vi "Logging Loop.vi"(5 "Acquisition and Logging":refnum<queue>, 7 "Message Handler":refnum<queue>, 8 "FIFO Cluster":T1, 9 "Name Cluster":T2, 10 "Ready to log":refnum<vi>, 11 "Logging Cluster":refnum<vi>) -> ()   [LabVIEW 2017]
uses:
  Controls/Logging names.ctl
  Message Queue/Message Cluster.ctl
  Message Queue/Message Queue.lvlib
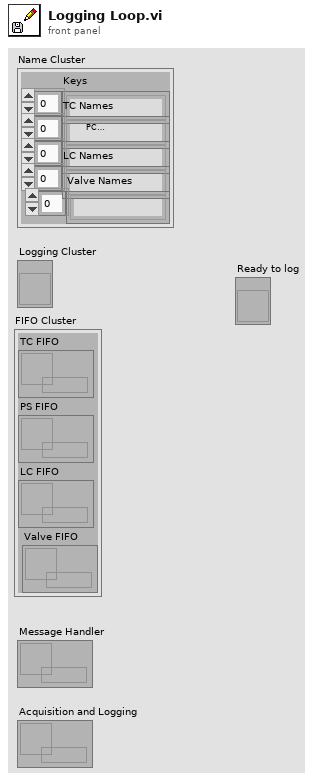
[diagram p1: front panel]
types:
  T1 = cluster{"TC FIFO":refnum<k33>, "PS FIFO":refnum<k33>, "LC FIFO":refnum<k33>, "Valve FIFO":refnum<k33>}
  T2 = typedef "Logging names.ctl" = cluster{"Keys":string[], "TC Names":string[], "PC Names":string[], "LC Names":string[], "Valve Names":string[]}
  T3 = cluster{"TC Logging":cluster{"TC 1":bool, "TC 2":bool, "TC 3":bool, "TC 4":bool, "TC 5":bool, "TC 6":bool, "TC 7":bool, "TC 8":bool, "TC 9":bool, "TC 10":bool, "TC 11":bool, "TC 12":bool, "TC 13":bool, "TC 14":bool, "TC 15":bool, "TC 16":bool}, "PS Logging":cluster{"PS 1":bool, "PS 2":bool, "PS 3":bool, "PS 4":bool, "PS 5":bool, "PS 6":bool, "PS 7":bool, "PS 8":bool}, "LC Logging":cluster{"LC 1":bool, "LC 2":bool, "LC 3":bool, "LC 4":bool}}
  T4 = enum16{"open", "open or create", "create or replace", "create", "open (read-only)"}
  T5 = typedef "Logging Settings.ctl" = cluster{"Logging Channels":cluster{"TC Logging":cluster{"TC 1":bool, "TC 2":bool, "TC 3":bool, "TC 4":bool, "TC 5":bool, "TC 6":bool, "TC 7":bool, "TC 8":bool, "TC 9":bool, "TC 10":bool, "TC 11":bool, "TC 12":bool, "TC 13":bool, "TC 14":bool, "TC 15":bool, "TC 16":bool}, "PS Logging":cluster{"PS 1":bool, "PS 2":bool, "PS 3":bool, "PS 4":bool, "PS 5":bool, "PS 6":bool, "PS 7":bool, "PS 8":bool}, "LC Logging":cluster{"LC 1":bool, "LC 2":bool, "LC 3":bool, "LC 4":bool}}, "TC Low Speed Logging":u32, "TC  High Speed Logging":u32, "PS Low Speed Logging":u32, "PS  High Speed Logging":u32, "LC Low Speed Logging":u32, "LC  High Speed Logging":u32, "Valve Names":string[]}
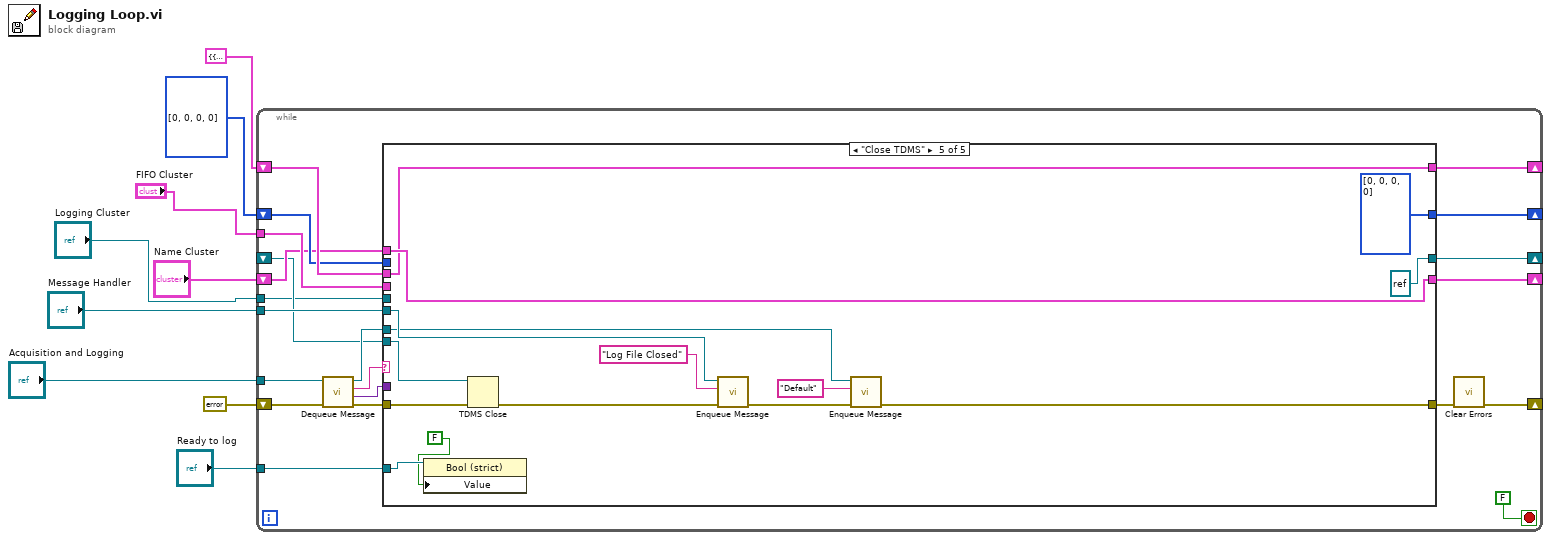
[diagram p0: block diagram]
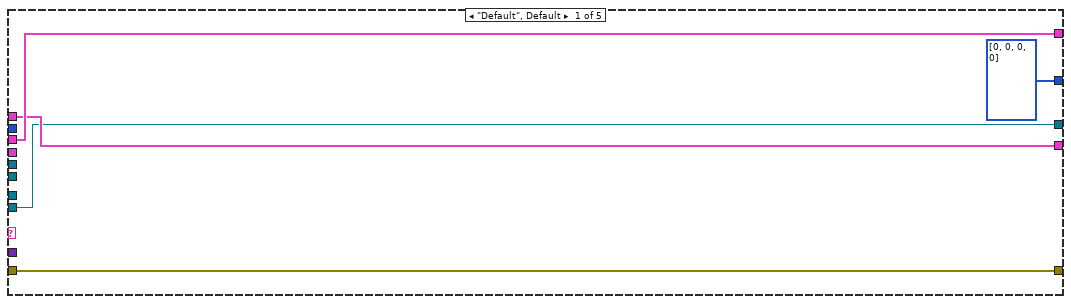
[diagram p2: hidden frame]
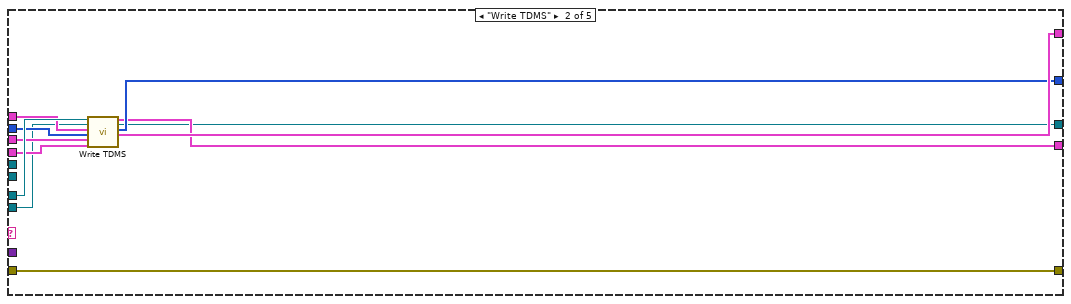
[diagram p3: hidden frame]
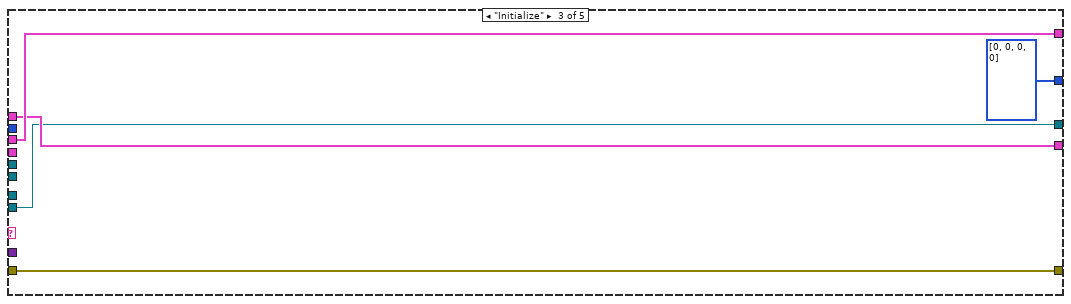
[diagram p4: hidden frame]
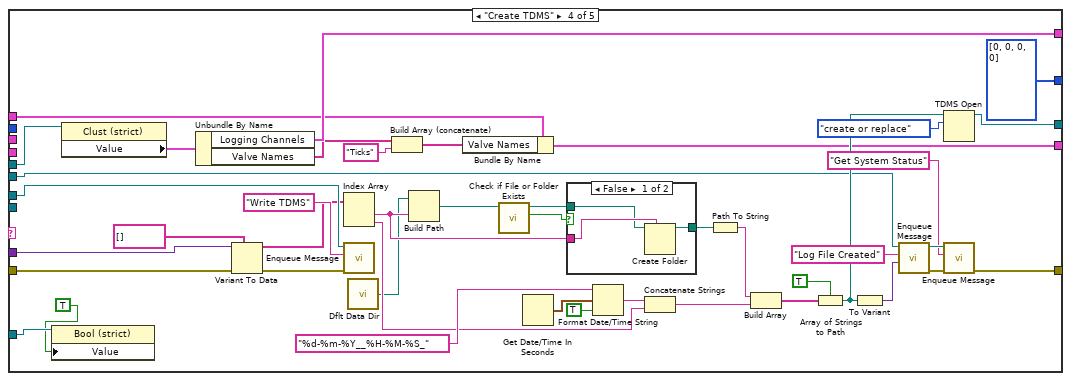
[diagram p5: hidden frame]
diagram:
  n1 = while {
    tunnel: "Acquisition and Logging" -> [w30]
    shift-right: [w18] -> _
    shift-left: errorcluster {"status"=FALSE, "code"=0, "source"=""} ("error out") -> [w24]
    tunnel: "FIFO Cluster" -> [w22]
    tunnel: "Message Handler" -> [w21]
    shift-right: [w20] -> _
    shift-left: T3 {"TC Logging"={"TC 1"=FALSE, "TC 2"=FALSE, "TC 3"=FALSE, "TC 4"=FALSE, "TC 5"=FALSE, "TC 6"=FALSE, "TC 7"=FALSE, "TC 8"=FALSE, "TC 9"=FALSE, "TC 10"=FALSE, "TC 11"=FALSE, "TC 12"=FALSE, "TC 13"=FALSE, "TC 14"=FALSE, "TC 15"=FALSE, "TC 16"=FALSE}, "PS Logging"={"PS 1"=FALSE, "PS 2"=FALSE, "PS 3"=FALSE, "PS 4"=FALSE, "PS 5"=FALSE, "PS 6"=FALSE, "PS 7"=FALSE, "PS 8"=FALSE}, "LC Logging"={"LC 1"=FALSE, "LC 2"=FALSE, "LC 3"=FALSE, "LC 4"=FALSE}} ("Logging Channels") -> [w19]
    shift-right: [w16] -> _
    shift-left: u32[] [0, 0, 0, 0] -> [w17]
    shift-right: [w15] -> _
    shift-left: "Name Cluster" -> [w14]
    shift-right: [w13] -> _
    shift-left: _ -> [w12]
    tunnel: "Logging Cluster" -> [w11]
    tunnel: "Ready to log" -> [w10]
    stop <- FALSE stop-if-true
    n2 = call "Dequeue Message.vi"("error in (no error)"=w24, "Message Queue"=w30) -> ("error out"=w29:errorcluster, "Message Data"=w27:variant, "Message"=w26:string, "dup Message Queue"=w28:refnum<queue>)  [unwired: 6 in]
    n3 = case shown="\"Close TDMS\"" w26 {
      tunnel: w29 -> [w35 w46 w48 w81 w113]
      tunnel: w28 -> [_ w45 _ w89 w104]
      tunnel: w27 -> [_ _ _ w82 _]
      tunnel: [w35 w46 w48 w66 w105] -> w23
      tunnel: w22 -> [_ w43 _ _ _]
      tunnel: w14 -> [w32 w44 w49 w76 w112]
      tunnel: w21 -> [_ _ _ w69 w109]
      tunnel: [w34 w40 w51 w84 w111] -> w20
      tunnel: w19 -> [w34 w42 w51 _ w111]
      tunnel: w17 -> [_ w41 _ _ _]
      tunnel: [u32[] [0, 0, 0, 0] w39 u32[] [0, 0, 0, 0] u32[] [0, 0, 0, 0] u32[] [0, 0, 0, 0]] -> w16
      tunnel: [w32 w38 w49 w73 w112] -> w15
      tunnel: [w31 w37 w47 w65 refnum<k34> refnum ("tdms file out")] -> w13
      tunnel: w12 -> [w31 w36 w47 _ w101]
      tunnel: w11 -> [_ _ _ w64 _]
      tunnel: w10 -> [_ _ _ w53 w100]
      frame "Default", Default {
      }
      frame "Write TDMS" {
        n4 = call "Write TDMS.vi"("Queue In"=w45, "TDMS File In"=w36, "TDMS Group Names"=w44, "Elements Remaning"=w41, "Logging Channel Cluster"=w42, "FIFO Cluster"=w43) -> (14:"Logging Channel Cluster"=w38:T2, "TDMS Out"=w37:refnum<k34>, "Elements Remaining Out"=w39:u32[], 17:"Logging Channel Cluster"=w40:T3)  [unwired: 10 in]
      }
      frame "Initialize" {
      }
      frame "Create TDMS" {
        n5 = property class="Bool (strict)"(reference=w53, "Value"=TRUE ("Ready to log")) -> ()  [unwired: 1 in, 2 out]
        n6 = property class="Clust (strict)"(reference=w64) -> ("Value"=w72:T5)  [unwired: 1 in, 2 out]
        n7 = Unbundle By Name(w72) -> ("Logging Channels"=w84:T3, "Valve Names"=w71:string[])
        n8 = Variant To Data(error in=w81, type=string[] [], Variant=w82) -> (data=w62:string[], error out=w80:errorcluster)
        n9 = Index Array(array=w62) -> (element #1=w57:string, element #2=w61:string)  [unwired: 2 in]
        n10 = call "Enqueue Message.vi"("error in (no error)"=w80, "Message"="Write TDMS", "Message Queue"=w89) -> ()  [unwired: 7 in, 2 out]
        n11 = call <vilib>:"Dflt Data Dir.vi"() -> ("App:Default Data Directory"=w55:path)
        n12 = Build Array (concatenate)(w71, "Ticks") -> (w74:string[])
        n13 = Build Path(base path=w55, name or relative path=w57) -> (appended path=w59:path)
        n14 = Bundle By Name(cluster=w76, "Valve Names"=w74) -> (w73:T2)
        n15 = call <vilib>:"Check if File or Folder Exists.vi"("path"=w59) -> ("file or folder exists?"=w58:bool, "dup path"=w54:path)  [unwired: 8 in, 1 out]
        n16 = Get Date/Time In Seconds() -> (seconds since 1Jan1904=w94:timestamp)
        n17 = case shown="False" w58 {
          tunnel: w57 -> [w97 _]
          tunnel: [w96 w98] -> w56
          tunnel: w54 -> [w95 w98]
          frame False {
            n18 = Create Folder(prompt (Create Folder)=w97, path (use dialog)=w95) -> (created path=w96:path)  [unwired: 1 in, 2 out]
          }
          frame True {
          }
        }
        n19 = Format Date/Time String(time format string (%c)="%d-%m-%Y__%H-%M-%S_", seconds (now)=w94, UTC format=TRUE) -> (date/time string=w90:string)
        n20 = Concatenate Strings(w90, w61) -> (w83:string)
        n21 = Path To String(path=w56) -> (string=w60:string)
        n22 = Build Array(w60, w83) -> (w86:string[])
        n23 = Array of Strings to Path(0:w86, 1:TRUE ("relative")) -> (2:w79:path)
        n24 = To Variant(anything=w79) -> (Variant=w87:variant)
        n25 = call "Enqueue Message.vi"("Message Data"=w87, "Message"="Log File Created", "Message Queue"=w69) -> ("error out"=w70:errorcluster, "dup Message Queue"=w68:refnum<queue>)  [unwired: 7 in]
        n26 = TDMS Open(10:T4."create or replace" ("operation (0:open)"), 11:w79) -> (3:w65:refnum<k34>)  [unwired: 5 in, 1 out]
        n27 = call "Enqueue Message.vi"("error in (no error)"=w70, "Message"="Get System Status", "Message Queue"=w68) -> ("error out"=w66:errorcluster)  [unwired: 7 in, 1 out]
      }
      frame "Close TDMS" {
        n28 = property class="Bool (strict)"(reference=w100, "Value"=FALSE ("Ready to log")) -> ()  [unwired: 1 in, 2 out]
        n29 = TDMS Close(8:w113, 11:w101) -> (0:w107:errorcluster)  [unwired: 1 out]
        n30 = call "Enqueue Message.vi"("error in (no error)"=w107, "Message"="Log File Closed", "Message Queue"=w109) -> ("error out"=w106:errorcluster)  [unwired: 7 in, 1 out]
        n31 = call "Enqueue Message.vi"("error in (no error)"=w106, "Message"="Default", "Message Queue"=w104) -> ("error out"=w105:errorcluster)  [unwired: 7 in, 1 out]
      }
    }
    n32 = call <vilib>:"Clear Errors.vi"("error in (no error)"=w23) -> ("error out"=w18:errorcluster)  [unwired: 5 in, 1 out]
  }
